vi "SWERVE DRIVE one corner.vi"(0 "swerve mod\ndata":T17 {"swerve STEER motor"."gear ratio" format="%_5f"; "swerve STEER motor"."MOTOR SELECT" items=["REV NEO"=5676, "REV NEO 550"=11000, "VEX Falcon"=6380, "WC Kraken"=6000]; "swerve DRIVE motor"."gear ratio" format="%_5f"; "swerve DRIVE motor"."MOTOR SELECT" items=["REV NEO"=5676, "REV NEO 550"=11000, "VEX Falcon"=6380, "WC Kraken"=6000]; "swerve module"."corner wt (lbm)" format="%_4f"; "swerve module"."POS" format="%.3g"; "swerve module"."coord wrt geom CTR"."Y" format="%.4g"; "swerve module"."coord wrt geom CTR"."X" format="%.4g"; "swerve module"."from pivot to module"."theta park (deg)" format="%.4g"; "swerve module"."from pivot to module"."theta spin (deg)" format="%.4g"; "swerve module"."from pivot to module"."theta (deg)" format="%.4g"; "swerve module"."from pivot to module"."R" format="%.4g"; "swerve module"."ABS" format="%.3g"; "swerve module"."target" format="%.3g"; "swerve module"."V" format="%.3g"}, 2 "distance (ft)":dbl, 3 "Control Mode":T18 items=["PercentOutput"=0, "Position"=1, "Velocity"=2, "Current"=3, "Follower"=5, "MotionProfile"=6, "MotionMagic"=7, "MotionProfileArc"=10, "Disabled"=15], 5 "error in (no error)":errorcluster) -> (13 "swerve module out":T10 {"corner wt (lbm)" format="%_4f"; "POS" format="%.3g"; "coord wrt geom CTR"."Y" format="%.4g"; "coord wrt geom CTR"."X" format="%.4g"; "from pivot to module"."theta park (deg)" format="%.4g"; "from pivot to module"."theta spin (deg)" format="%.4g"; "from pivot to module"."theta (deg)" format="%.4g"; "from pivot to module"."R" format="%.4g"; "ABS" format="%.3g"; "target" format="%.3g"; "V" format="%.3g"}, 14 "velocity out":dbl, 15 "steer angle out\n(deg)":dbl, 19 "error out":errorcluster)   [LabVIEW 2023]
uses:
  <vilib>/Rock Robotics/WPI/ThirdParty/Phoenix-LabVIEW/CANCoder/Get/CTRE_Phoenix_CANcoder_GetSensorData.vi
  <vilib>/Rock Robotics/WPI/ThirdParty/REV Robotics/REVLib/SubVI/Public/SPARK Get Device Status Output Current.vi
  ctrl defs/ctrl Spark MAX current limiting.ctl
  <vilib>/Rock Robotics/WPI/ThirdParty/REV Robotics/REVLib/Typedef/Spark MAX Idle Mode.ctl
  ctrl defs/ctrl MOTOR SELECT.ctl
  <vilib>/Rock Robotics/WPI/ThirdParty/REV Robotics/REVLib/Typedef/Spark MAX Smart Motion Parameters.ctl
  ctrl defs/ctrl motor PIDF coefficients.ctl
  ctrl defs/ctrl swerve motor.ctl
  <vilib>/Rock Robotics/SystemInterfaces/DIO/FPGA_DIOPWMChannel.ctl
  <vilib>/Rock Robotics/WPI/PWM/WPI_PWMDeadband.ctl
  <vilib>/Rock Robotics/WPI/MotorControl/WPI_MotorControlType.ctl
  <vilib>/Rock Robotics/SystemInterfaces/DIO/FPGA_DIOChannel.ctl
  <vilib>/Rock Robotics/WPI/MotorControl/WPI_MotorControlDeviceRef.ctl
  <vilib>/Rock Robotics/WPI/ThirdParty/Phoenix-LabVIEW/CANCoder/Controls/CTRE_Phoenix_CANcoder_DeviceRef.ctl
  ctrl defs/ctrl swerve module.ctl
  <vilib>/Rock Robotics/WPI/ThirdParty/Phoenix-LabVIEW/Motor Controller/Controls/CTRE_Phoenix_MotorControl_ControlMode.ctl
  <vilib>/Rock Robotics/WPI/ThirdParty/Phoenix-LabVIEW/Motor Controller/Controls/CTRE_Phoenix_MotorControl_TalonFXInvertType.ctl
  <vilib>/Rock Robotics/WPI/ThirdParty/Phoenix-LabVIEW/Motor Controller/Controls/CTRE_Phoenix_MotorControl_NeutralMode.ctl
  ctrl defs/ctrl Talon FX config.ctl
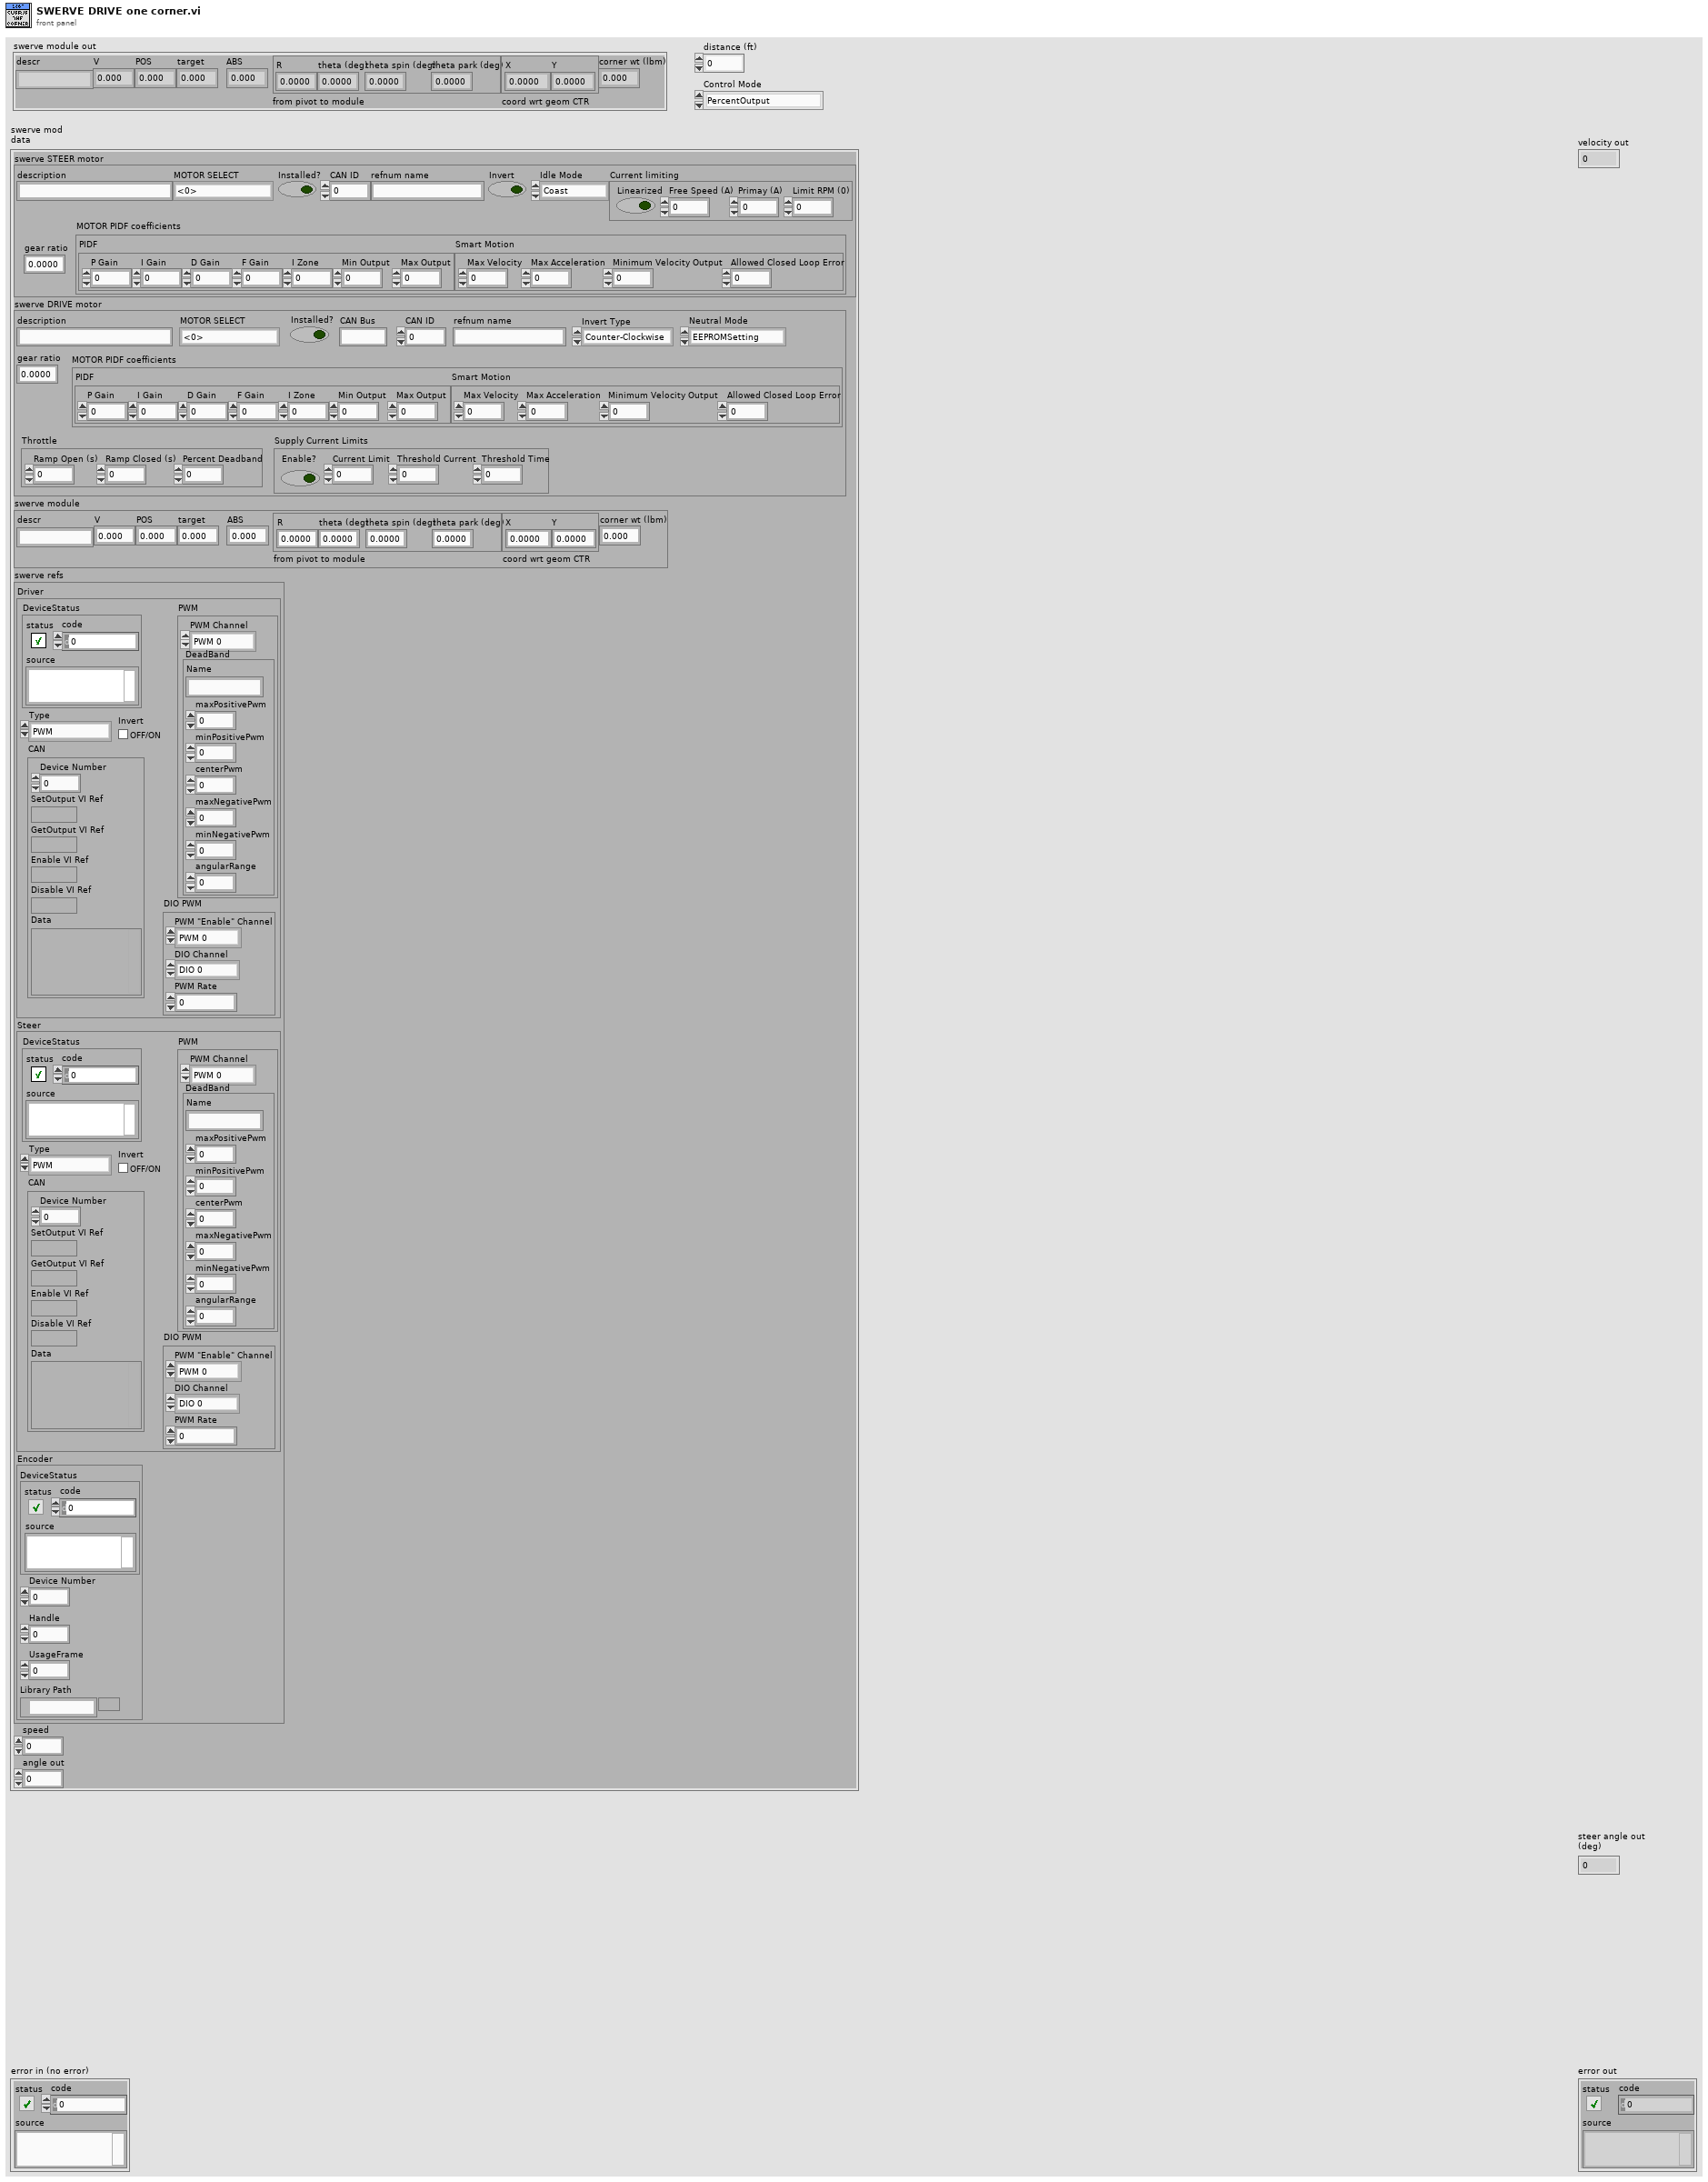
[diagram p1: front panel]
types:
  T1 = typedef "ctrl swerve motor.ctl" = cluster{"description":string, "MOTOR SELECT":T2, "Installed?":bool, "CAN ID":u8, "refnum name":string, "Invert":bool, "Idle Mode":T3, "Current limiting":T4, "MOTOR PIDF coefficients":T5, "gear ratio":dbl}
  T2 = typedef "ctrl MOTOR SELECT.ctl" = i16
  T3 = typedef "Spark MAX Idle Mode.ctl" = enum16{"Coast", "Brake"}
  T4 = typedef "ctrl Spark MAX current limiting.ctl" = cluster{"Linearized":bool, "Free Speed (A)":dbl, "Primay (A)":dbl, "Limit RPM (0)":u32}
  T5 = typedef "ctrl motor PIDF coefficients.ctl" = cluster{"PIDF":cluster{"P Gain":dbl, "I Gain":dbl, "D Gain":dbl, "F Gain":dbl, "I Zone":dbl, "Min Output":dbl, "Max Output":dbl}, "Smart Motion":T6}
  T6 = typedef "Spark MAX Smart Motion Parameters.ctl" = cluster{"Max Velocity":dbl, "Max Acceleration":dbl, "Minimum Velocity Output":dbl, "Allowed Closed Loop Error":dbl}
  T7 = typedef "ctrl Talon FX config.ctl" = cluster{"refnum name":string, "CAN ID":u8, "Installed?":bool, "description":string, "MOTOR SELECT":T2, "CAN Bus":string, "Invert Type":T8, "Neutral Mode":T9, "gear ratio":dbl, "MOTOR PIDF coefficients":T5, "Throttle":cluster{"Ramp Open (s)":dbl, "Ramp Closed (s)":dbl, "Percent Deadband":dbl}, "Supply Current Limits":cluster{"Enable?":bool, "Current Limit":dbl, "Threshold Current":dbl, "Threshold Time":dbl}}
  T8 = typedef "CTRE_Phoenix_MotorControl_TalonFXInvertType.ctl" = enum16{"Counter-Clockwise", "Clockwise"}
  T9 = typedef "CTRE_Phoenix_MotorControl_NeutralMode.ctl" = enum8{"EEPROMSetting", "Override to Coast", "Override to Brake"}
  T10 = typedef "ctrl swerve module.ctl" = cluster{"descr":string, "V":dbl, "POS":dbl, "target":dbl, "ABS":dbl, "from pivot to module":cluster{"R":dbl, "theta (deg)":dbl, "theta spin (deg)":dbl, "theta park (deg)":dbl}, "coord wrt geom CTR":cluster{"X":dbl, "Y":dbl}, "corner wt (lbm)":dbl}
  T11 = typedef "WPI_MotorControlDeviceRef.ctl" = cluster{"DeviceStatus":errorcluster, "Type":T12, "PWM":cluster{"PWM Channel":T13, "DeadBand":T14}, "CAN":cluster{"Device Number":u8, "SetOutput VI Ref":variant, "GetOutput VI Ref":variant, "Enable VI Ref":variant, "Disable VI Ref":variant, "Data":variant}, "Invert":bool, "DIO PWM":cluster{"PWM \"Enable\" Channel":T13, "DIOChannel":T15, "PWM Rate":dbl}}
  T12 = typedef "WPI_MotorControlType.ctl" = enum16{"PWM", "CAN", "DIO PWM"}
  T13 = typedef "FPGA_DIOPWMChannel.ctl" = enum8{"PWM 0", "PWM 1", "PWM 2", "PWM 3", "PWM 4", "PWM 5", "PWM 6", "PWM 7", "PWM 8", "PWM 9", "PWM MXP 0", "PWM MXP 1", "PWM MXP 2", "PWM MXP 3", "PWM MXP 4", "PWM MXP 5", "PWM MXP 6", "PWM MXP 7", "PWM MXP 8", "PWM MXP 9", "Invalid"}
  T14 = typedef "WPI_PWMDeadband.ctl" = cluster{"Name":string, "maxPositivePwm":i32, "minPositivePwm":i32, "centerPwm":i32, "maxNegativePwm":i32, "minNegativePwm":i32, "angularRange":u16}
  T15 = typedef "FPGA_DIOChannel.ctl" = enum8{"DIO 0", "DIO 1", "DIO 2", "DIO 3", "DIO 4", "DIO 5", "DIO 6", "DIO 7", "DIO 8", "DIO 9", "DIO MXP 0", "DIO MXP 1", "DIO MXP 2", "DIO MXP 3", "DIO MXP 4", "DIO MXP 5", "DIO MXP 6", "DIO MXP 7", "DIO MXP 8", "DIO MXP 9", "DIO MXP 10", "DIO MXP 11", "DIO MXP 12", "DIO MXP 13", "DIO MXP 14", "DIO MXP 15", "SPI Port CS1", "SPI Port CS2", "SPI Port CS3", "SPI Port MISO", "SPI Port MOSI", "Invalid"}
  T16 = typedef "CTRE_Phoenix_CANcoder_DeviceRef.ctl" = cluster{"DeviceStatus":errorcluster, "Device Number":u8, "Handle":u64, "UsageFrame":u32, "Library Path":path}
  T17 = cluster{"swerve STEER motor":T1, "swerve DRIVE motor":T7, "swerve module":T10, "swerve refs":cluster{"Driver":T11, "Steer":T11, "Encoder":T16}, "speed":dbl, "angle out":dbl}
  T18 = typedef "CTRE_Phoenix_MotorControl_ControlMode.ctl" = u16
  T19 = cluster{"Driver":T11, "Steer":T11, "Encoder":T16}
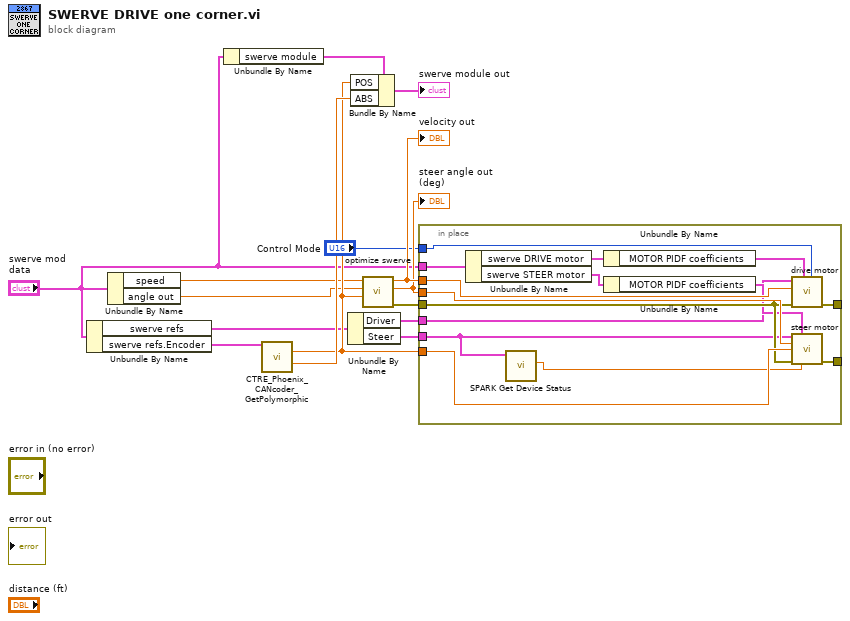
[diagram p0: block diagram]
diagram:
  n1 = Unbundle By Name("swerve mod\ndata") -> ("swerve refs"=w5:T19, "swerve refs.Encoder"=w6:T16)
  n2 = Unbundle By Name("swerve mod\ndata") -> ("speed"=w2:dbl, "angle out"=w3:dbl)
  n3 = Unbundle By Name("swerve mod\ndata") -> ("swerve module"=w4:T10)
  n4 = call-poly <vilib>:"CTRE_Phoenix_CANcoder_GetPolymorphic.vi"("CTRE_CANcoder_DeviceRef"=w6) -> ("Position"=w10:dbl, "Absolute Position"=w11:dbl)  [unwired: 10 in, 3 out]
  n5 = Unbundle By Name(w5) -> ("Driver"=w12:T11, "Steer"=w8:T11)
  n6 = Bundle By Name(cluster=w4, "POS"=w10, "ABS"=w11) -> (→"swerve module out":T10)
  n7 = call "optimize swerve.vi"("current angle (deg)"=w10, "target angle (deg)"=w3, "velocity"=w2) -> ("error out"=w13:errorcluster, "steer angle (deg)"=w14:dbl, "velocity"=w15:dbl)  [unwired: 5 in, 1 out]
  "velocity out" <- w15
  "steer angle out\n(deg)" <- w14
  n8 = in-place {
    in-place-border: w14 -> [w30]
    in-place-border: w8 -> [w19]
    in-place-border: w10 -> [w29]
    in-place-border: w12 -> [w21]
    in-place-border: w15 -> [w28]
    in-place-border: w13 -> [w27]
    in-place-border: [w26] -> _
    in-place-border: [w25] -> _
    in-place-border: "Control Mode" -> [w22]
    in-place-border: "swerve mod\ndata" -> [w16]
    n9 = Unbundle By Name(w16) -> ("swerve DRIVE motor"=w18:T7, "swerve STEER motor"=w17:T1)
    n10 = call-poly <vilib>:"SPARK Get Device Status.vi"("MotorControlDevRef in"=w19) -> ("Current"=w20:dbl)  [unwired: 7 in, 3 out]
    n11 = Unbundle By Name(w18) -> ("MOTOR PIDF coefficients"=w24:T5)
    n12 = Unbundle By Name(w17) -> ("MOTOR PIDF coefficients"=w23:T5)
    n13 = call "drive motor.vi"("Control Mode"=w22, "MOTOR PIDF coefficients"=w24, "error in (no error)"=w27, "velocity"=w28, "Driver"=w21) -> ("error out"=w26:errorcluster)  [unwired: 6 in]
    n14 = call "steer motor.vi"("MotorControlDevRef"=w19, "MOTOR PIDF coefficients"=w23, "target"=w30, "encoder"=w29, "error in (no error)"=w27, "DRIVE motor\ncurrent (A)"=w20) -> ("error out"=w25:errorcluster)  [unwired: 9 in]
  }
